vi "oa_Draw Clearance Boundary for SCL Plot.vi"(5 "shaft center line settings":T3={"cartesian grid cosmetics"={"line color"=39168, "text color"=65280, "tick length(3)"=3, "crossing axes"=FALSE, "visible grid?"=TRUE}, "XY plot cosmetics"={"plot color"=16776960, "XY plot type"=enum."connected points", "baseline"=0.0}, "desired font(Application)"=enum."Application Font", "[user-specified font]"={"Font Name:"="", "Size"=0, "Strikeout?"=FALSE, "Italic?"=FALSE, "Underline?"=FALSE, "Outline?"=FALSE, "Shadow?"=FALSE, "Bold?"=FALSE}} {"XY plot cosmetics"."baseline" format="%0.2f"}, 6 "clearance boundary settings":T1={"start point"=enum."center", " boundary"={"x axis"=0.0, "y axis"=0.0}}, 8 "error in (no error)":errorcluster, 9 "y scale factors":cluster{"a":dbl, "b":dbl, "log?":bool} {"b" format="%0.2f"; "a" format="%0.2f"}, 10 "x scale factors":cluster{"a":dbl, "b":dbl, "log?":bool} {"b" format="%0.2f"; "a" format="%0.2f"}, 11 "picture":picture) -> (0 "error out":errorcluster, 3 "new picture":picture)   [LabVIEW 2017]
uses:
  <vilib>/picture/cartesn2.llb/XY Plot Type.ctl
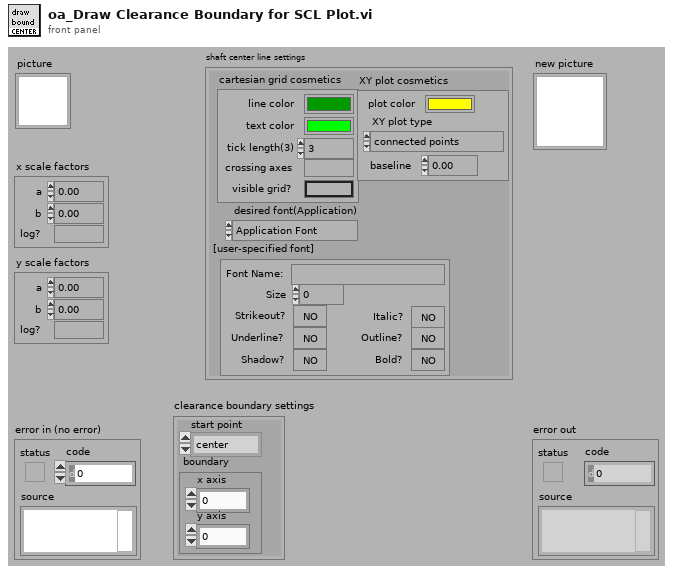
[diagram p1: front panel]
types:
  T1 = cluster{"start point":enum16{"top", "center", "bottom"}, " boundary":cluster{"x axis":dbl, "y axis":dbl}}
  T2 = typedef "XY Plot Type.ctl" = enum16{"points", "squares", "circles", "connected points", "connected squares", "connected circles", "comb plot", "sized scatter plot", "sized-colored scatter plot", "min-max lines"}
  T3 = cluster{"cartesian grid cosmetics":cluster{"line color":u32, "text color":u32, "tick length(3)":i16, "crossing axes":bool, "visible grid?":bool}, "XY plot cosmetics":cluster{"plot color":u32, "XY plot type":T2, "baseline":dbl}, "desired font(Application)":enum16{"User-specified Font", "Application Font", "System Font", "Dialog Font"}, "[user-specified font]":cluster{"Font Name:":string, "Size":i16, "Strikeout?":bool, "Italic?":bool, "Underline?":bool, "Outline?":bool, "Shadow?":bool, "Bold?":bool}}
  T4 = cluster{"Width":u16, "Style":enum32{"Solid", "Dash", "Dot", "DashDot", "DashDotDot"}}
  T5 = cluster{"line color":u32, "text color":u32, "tick length(3)":i16, "crossing axes":bool, "visible grid?":bool}
  T6 = cluster{"pixel":dbl, "pixel":dbl, "pixel":dbl, "pixel":dbl}
  T7 = cluster{"pixel":i16, "pixel":i16, "pixel":i16, "pixel":i16}
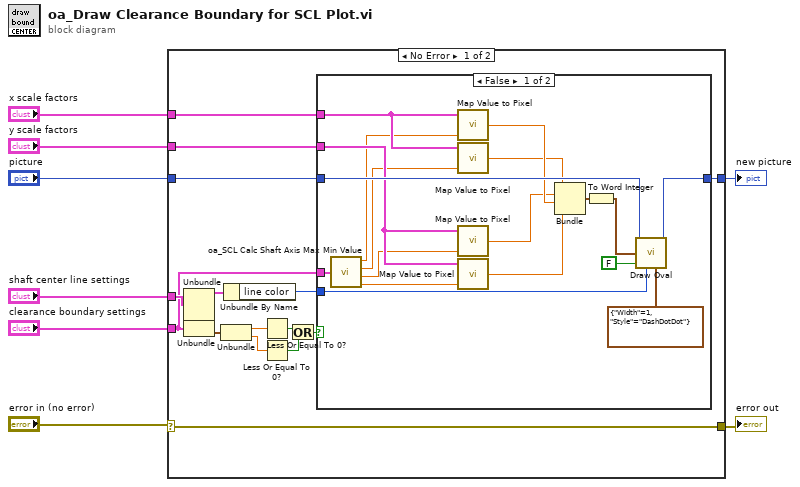
[diagram p0: block diagram]
diagram:
  n1 = case shown="No Error" "error in (no error)" {
    selector: "error in (no error)" -> [w23 w44]
    tunnel: [w23 w44] -> w7
    tunnel: "clearance boundary settings" -> [w10 _]
    tunnel: "picture" -> [w18 w43]
    tunnel: [w17 w43] -> w4
    tunnel: "shaft center line settings" -> [w16 _]
    tunnel: "x scale factors" -> [w14 _]
    tunnel: "y scale factors" -> [w13 _]
    frame No Error {
      n2 = Unbundle(w16) -> ("cartesian grid cosmetics"=w9:T5)  [unwired: 3 out]
      n3 = Unbundle(w10) -> ("boundary"=w22:cluster{"x axis":dbl, "y axis":dbl})  [unwired: 1 out]
      n4 = Unbundle(w22) -> ("x axis"=w12:dbl, "y axis"=w11:dbl)
      n5 = Unbundle By Name(w9) -> ("line color"=w15:u32)
      n6 = Less Or Equal To 0?(x=w12) -> (x <= 0?=w21:bool)
      n7 = Less Or Equal To 0?(x=w11) -> (x <= 0?=w20:bool)
      n8 = Or(x=w21, y=w20) -> (x .or. y?=w19:bool)
      n9 = case shown="False" w19 {
        tunnel: w18 -> [w38 w42]
        tunnel: [w37 w42] -> w17
        tunnel: w15 -> [w41 _]
        tunnel: w14 -> [w35 _]
        tunnel: w13 -> [w34 _]
        tunnel: w10 -> [w36 _]
        frame False {
          n10 = call <vilib>:"oa_SCL Calc Shaft Axis Max Min Value.vi"("clearance boundary settings"=w36) -> ("x axis max"=w31:dbl, "x axis min"=w30:dbl, "y axis max"=w29:dbl, "y axis min"=w28:dbl)
          n11 = call <vilib>:"Map Value to Pixel.vi"("x"=w31, "scale factors"=w35) -> ("pixel"=w27:dbl)  [unwired: 1 in]
          n12 = call <vilib>:"Map Value to Pixel.vi"("x"=w30, "scale factors"=w35) -> ("pixel"=w26:dbl)  [unwired: 1 in]
          n13 = call <vilib>:"Map Value to Pixel.vi"("x"=w29, "scale factors"=w34) -> ("pixel"=w25:dbl)  [unwired: 1 in]
          n14 = call <vilib>:"Map Value to Pixel.vi"("x"=w28, "scale factors"=w34) -> ("pixel"=w24:dbl)  [unwired: 1 in]
          n15 = Bundle("pixel"=w26, "pixel"=w25, "pixel"=w27, "pixel"=w24) -> (w33:T6)  [unwired: 1 in]
          n16 = To Word Integer(number=w33) -> (16bit integer=w32:T7)
          n17 = call <vilib>:"Draw Oval.vi"("picture"=w38, "rect"=w32, "fill?(F)"=FALSE, "color(black)"=w41, "pen"=T4 {"Width"=1, "Style"=enum."DashDotDot"}) -> ("new picture"=w37:picture)  [unwired: 4 in]
        }
        frame True {
        }
      }
    }
    frame Error {
    }
  }
  "new picture" <- w4
  "error out" <- w7
